vi "%s (Request & Reply).vi"(7 "Additional Reply Message Queues (Default 0)":i32, 8 "error in (no error)":errorcluster, 11 "API out":refnum<class "Interface.lvclass">) -> (0 "error out":errorcluster, 3 "API out":refnum<class "Interface.lvclass">)   [LabVIEW 2018, in "Scripting.lvlib" / "Actor.lvlib" / "Interface.lvclass"]
uses:
  Interface.lvclass
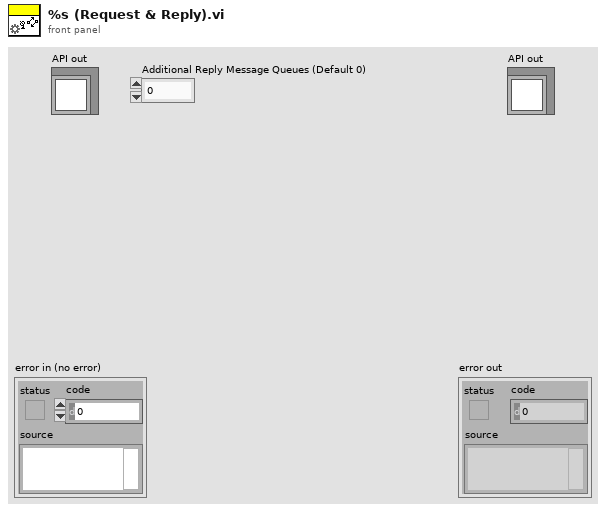
[diagram p1: front panel]
types:
  T1 = typedef "Scripting.lvlib/Actor.lvlib/Interface.lvclass/API-Data.ctl" = cluster{"Launch":refnum<notifier>, "Actor Stopped":cluster{"Enqueuer":refnum<user-event>, "Message":refnum<event-registration>}, "Requests":T2}
  T2 = typedef "Scripting.lvlib/Actor.lvlib/Actor.lvclass/Request-Enqueuers.ctl" = cluster{"Get State":refnum<user-event>, "Stop":refnum<user-event>}
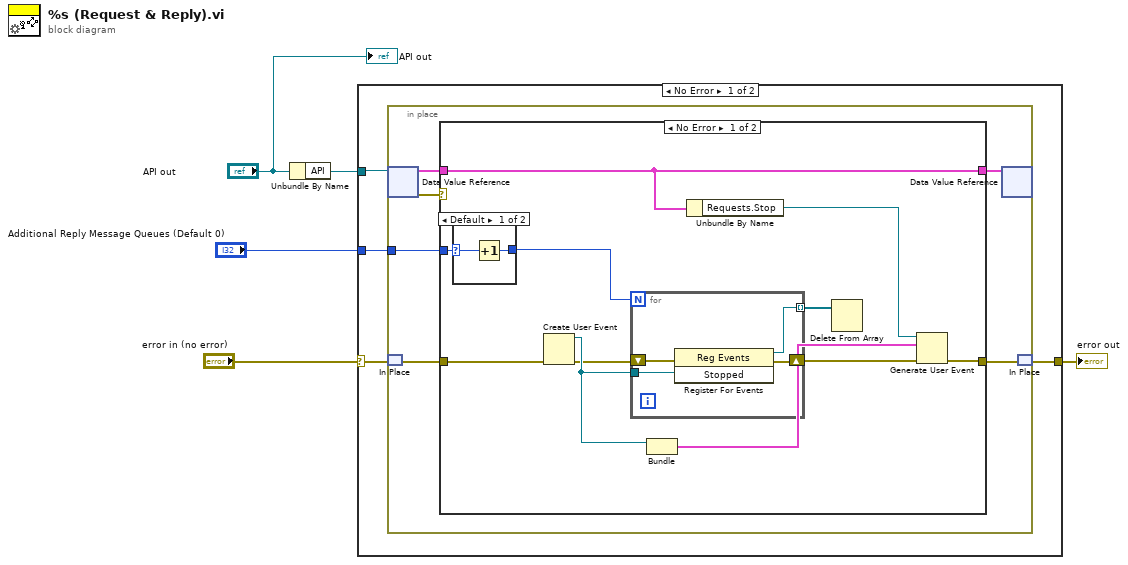
[diagram p0: block diagram]
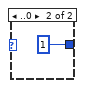
[diagram p2: hidden frame]
diagram:
  n1 = Unbundle By Name("API out") -> ("API"=w1:refnum<data-value>)
  n2 = case shown="No Error" "error in (no error)" {
    selector: "error in (no error)" -> [w9 w36]
    tunnel: [w8 w36] -> w4
    tunnel: w1 -> [w7 _]
    tunnel: "Additional Reply Message Queues (Default 0)" -> [w6 _]
    frame No Error {
      n3 = in-place {
        in-place-border: w6 -> [w10]
        n4 = in-place-dvr #1(w7) -> (w14:T1, w15:errorcluster)
        n5 = in-place-match #2(w9) -> (w12:errorcluster)
        n6 = case shown="No Error" w15 {
          selector: w15 -> [_ w35]
          tunnel: w14 -> [w26 w34]
          tunnel: [w26 w34] -> w13
          tunnel: w12 -> [w25 _]
          tunnel: [w23 w35] -> w11
          tunnel: w10 -> [w20 _]
          frame No Error {
            n7 = case shown="Default" w20 {
              selector: w20 -> [w28 _]
              tunnel: [w27 1] -> w19
              frame Default {
                n8 = Increment(x=w28) -> (x+1=w27:i32)
              }
              frame ..0 {
              }
            }
            n9 = Create User Event(error in=w25) -> (user event=w21:refnum<user-event>, error out=w18:errorcluster)  [unwired: 1 in]
            n10 = for {
              N: w19 -> [_]
              shift-right: [w32] -> w24
              shift-left: w18 -> [w33]
              tunnel: [w31] -> w17 mode=indexing
              tunnel: w21 -> [w30]
              n11 = register-events(error in=w33, w30) -> (reference out=w31:refnum<event-registration>, error out=w32:errorcluster)  [unwired: 1 in]
            }
            n12 = Bundle("Stopped"=w21) -> (w16:cluster{"Stopped":refnum<user-event>, void})  [unwired: 2 in]
            n13 = Unbundle By Name(w26) -> ("Requests.Stop"=w22:refnum<user-event>)
            n14 = Delete From Array(array=w17) -> ()  [unwired: 2 in, 2 out]
            n15 = Generate User Event(user event=w22, event data cluster=w16, error in=w24) -> (error out=w23:errorcluster)  [unwired: 1 in, 1 out]
          }
          frame Error {
          }
        }
        n16 = in-place-dvr #1(w13) -> ()  [unwired: 2 out]
        n17 = in-place-match #2(w11) -> (w8:errorcluster)
      }
    }
    frame Error {
    }
  }
  "error out" <- w4
  "API out" <- "API out"
